vi "Sensor checking_try.vi"() -> ()   [LabVIEW 2016]
uses:
  <vilib>/rvi/Emulation/niFpgaGetClockAttributes.vi
  <vilib>/rvi/Emulation/niFpgaSctlEmulationGetInTimedLoop.vi
  <vilib>/rvi/Emulation/niFpgaEmulationReportErrorSimple.vi
  <vilib>/rvi/eio/common/nirviEmuTemplateMethod_errors.vi
  <vilib>/rvi/Emulation/niFpgaCriticalErrorInLSC.vi
  <vilib>/eio/EIONode/EIONode.xnode
panel:
  out "8 9":fxp<+/-,26,5> format="%#_6f"
  out "8 8":fxp<+/-,26,5> format="%#_6f"
  out "8 7":fxp<+/-,26,5> format="%#_6f"
  out "8 6":fxp<+/-,26,5> format="%#_6f"
  out "8 5":fxp<+/-,26,5> format="%#_6f"
  out "8 4":fxp<+/-,26,5> format="%#_6f"
  out "8 3":fxp<+/-,26,5> format="%#_6f"
  out "8 2":fxp<+/-,26,5> format="%#_6f"
  out "8 1":fxp<+/-,26,5> format="%#_6f"
  out "7 9":fxp<+/-,26,5> format="%#_6f"
  out "7 8":fxp<+/-,26,5> format="%#_6f"
  out "7 7":fxp<+/-,26,5> format="%#_6f"
  out "7 6":fxp<+/-,26,5> format="%#_6f"
  out "7 5":fxp<+/-,26,5> format="%#_6f"
  out "7 4":fxp<+/-,26,5> format="%#_6f"
  out "7 3":fxp<+/-,26,5> format="%#_6f"
  out "7 2":fxp<+/-,26,5> format="%#_6f"
  out "7 1":fxp<+/-,26,5> format="%#_6f"
  out "6 9":fxp<+/-,26,5> format="%#_6f"
  out "6 8":fxp<+/-,26,5> format="%#_6f"
  out "6 7":fxp<+/-,26,5> format="%#_6f"
  out "6 6":fxp<+/-,26,5> format="%#_6f"
  out "6 5":fxp<+/-,26,5> format="%#_6f"
  out "6 4":fxp<+/-,26,5> format="%#_6f"
  out "6 3":fxp<+/-,26,5> format="%#_6f"
  out "6 2":fxp<+/-,26,5> format="%#_6f"
  out "6 1":fxp<+/-,26,5> format="%#_6f"
  out "5 9":fxp<+/-,26,5> format="%#_6f"
  out "5 8":fxp<+/-,26,5> format="%#_6f"
  out "5 7":fxp<+/-,26,5> format="%#_6f"
  out "5 6":fxp<+/-,26,5> format="%#_6f"
  out "5 5":fxp<+/-,26,5> format="%#_6f"
  out "5 4":fxp<+/-,26,5> format="%#_6f"
  out "5 3":fxp<+/-,26,5> format="%#_6f"
  out "5 2":fxp<+/-,26,5> format="%#_6f"
  out "5 1":fxp<+/-,26,5> format="%#_6f"
  out "4 9":fxp<+/-,26,5> format="%#_6f"
  out "4 8":fxp<+/-,26,5> format="%#_6f"
  out "4 7":fxp<+/-,26,5> format="%#_6f"
  out "4 6":fxp<+/-,26,5> format="%#_6f"
  out "4 5":fxp<+/-,26,5> format="%#_6f"
  out "4 4":fxp<+/-,26,5> format="%#_6f"
  out "4 3":fxp<+/-,26,5> format="%#_6f"
  out "4 2":fxp<+/-,26,5> format="%#_6f"
  out "4 1":fxp<+/-,26,5> format="%#_6f"
  out "3 9":fxp<+/-,26,5> format="%#_6f"
  out "3 8":fxp<+/-,26,5> format="%#_6f"
  out "3 7":fxp<+/-,26,5> format="%#_6f"
  out "3 6":fxp<+/-,26,5> format="%#_6f"
  out "3 5":fxp<+/-,26,5> format="%#_6f"
  out "3 4":fxp<+/-,26,5> format="%#_6f"
  out "3 3":fxp<+/-,26,5> format="%#_6f"
  out "3 2":fxp<+/-,26,5> format="%#_6f"
  out "3 1":fxp<+/-,26,5> format="%#_6f"
  out "2 9":fxp<+/-,26,5> format="%#_6f"
  out "2 8":fxp<+/-,26,5> format="%#_6f"
  out "2 7":fxp<+/-,26,5> format="%#_6f"
  out "2 6":fxp<+/-,26,5> format="%#_6f"
  out "2 5":fxp<+/-,26,5> format="%#_6f"
  out "2 4":fxp<+/-,26,5> format="%#_6f"
  out "2 3":fxp<+/-,26,5> format="%#_6f"
  out "2 2":fxp<+/-,26,5> format="%#_6f"
  out "2 1":fxp<+/-,26,5> format="%#_6f"
  out "1 9":fxp<+/-,26,5>
  out "1 8":fxp<+/-,26,5>
  out "1 7":fxp<+/-,26,5>
  out "1 6":fxp<+/-,26,5>
  out "1 5":fxp<+/-,26,5>
  out "1 4":fxp<+/-,26,5>
  out "1 3":fxp<+/-,26,5>
  out "1 2":fxp<+/-,26,5> format="%#_6f"
  out "1 1":fxp<+/-,26,5> format="%#_6f"
  in  "8":bool
  in  "7":bool
  in  "6":bool
  in  "5":bool
  in  "4":bool
  in  "3":bool
  in  "2":bool
  in  "1":bool
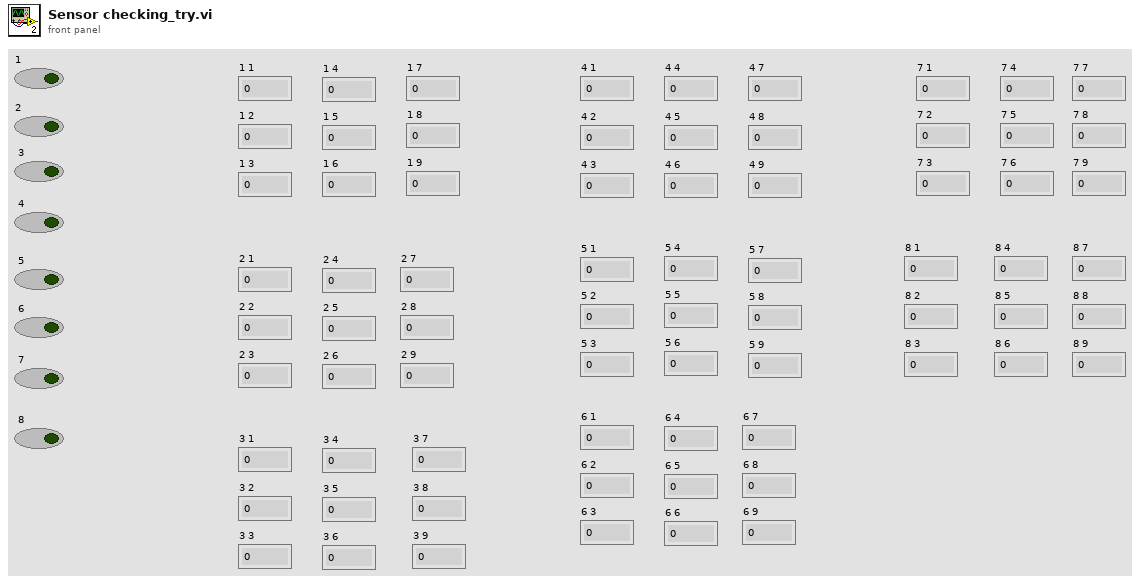
[diagram p1: front panel]
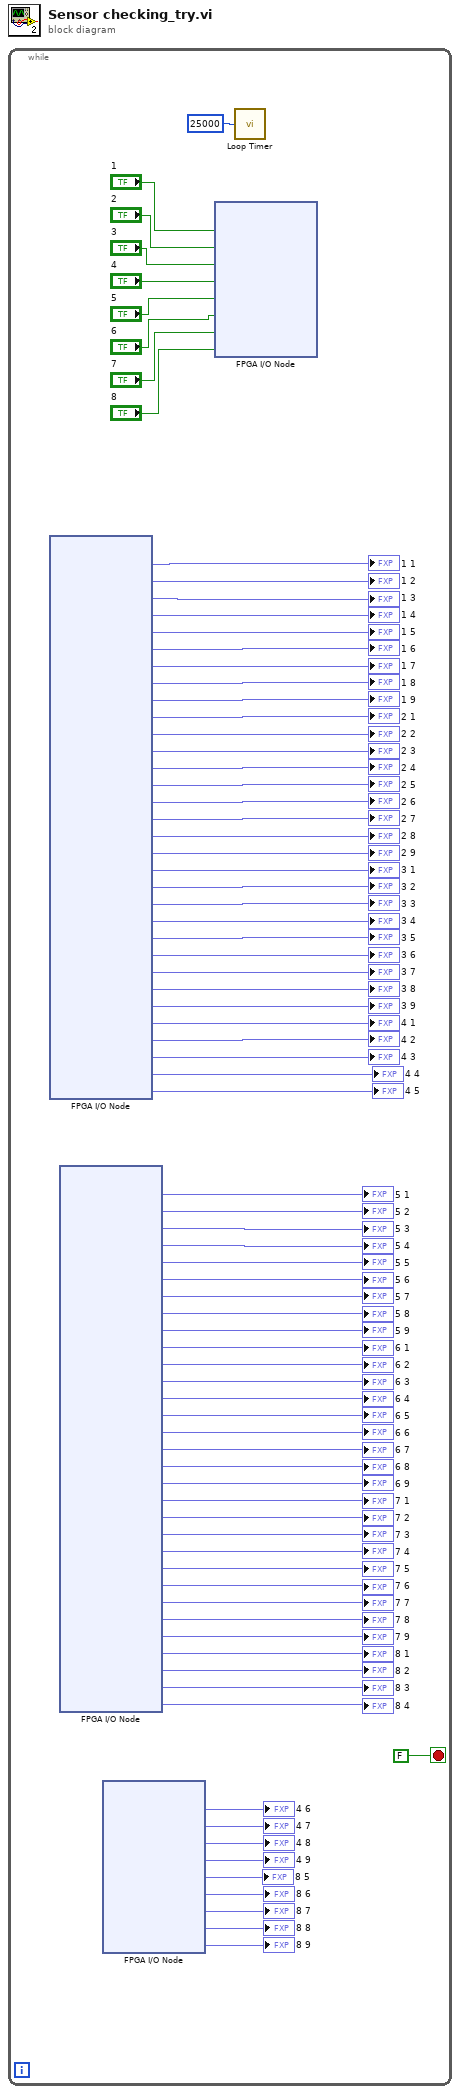
[diagram p0: block diagram]
diagram:
  n1 = while {
    stop <- FALSE stop-if-true
    n2 = xnode "FPGA I/O Node"() -> ("Mod1/AI0"=→"1 1":fxp<+/-,26,5>, "Mod1/AI1"=→"1 2":fxp<+/-,26,5>, "Mod1/AI2"=→"1 3":fxp<+/-,26,5>, "Mod1/AI3"=→"1 4":fxp<+/-,26,5>, "Mod1/AI4"=→"1 5":fxp<+/-,26,5>, "Mod1/AI5"=→"1 6":fxp<+/-,26,5>, "Mod1/AI6"=→"1 7":fxp<+/-,26,5>, "Mod1/AI7"=→"1 8":fxp<+/-,26,5>, "Mod1/AI8"=→"1 9":fxp<+/-,26,5>, "Mod1/AI9"=→"2 1":fxp<+/-,26,5>, "Mod1/AI10"=→"2 2":fxp<+/-,26,5>, "Mod1/AI11"=→"2 3":fxp<+/-,26,5>, "Mod1/AI12"=→"2 4":fxp<+/-,26,5>, "Mod1/AI13"=→"2 5":fxp<+/-,26,5>, "Mod1/AI14"=→"2 6":fxp<+/-,26,5>, "Mod1/AI15"=→"2 7":fxp<+/-,26,5>, "Mod1/AI16"=→"2 8":fxp<+/-,26,5>, "Mod1/AI17"=→"2 9":fxp<+/-,26,5>, "Mod1/AI18"=→"3 1":fxp<+/-,26,5>, "Mod1/AI19"=→"3 2":fxp<+/-,26,5>, "Mod1/AI20"=→"3 3":fxp<+/-,26,5>, "Mod1/AI21"=→"3 4":fxp<+/-,26,5>, "Mod1/AI22"=→"3 5":fxp<+/-,26,5>, "Mod1/AI23"=→"3 6":fxp<+/-,26,5>, "Mod1/AI24"=→"3 7":fxp<+/-,26,5>, "Mod1/AI25"=→"3 8":fxp<+/-,26,5>, "Mod1/AI26"=→"3 9":fxp<+/-,26,5>, "Mod1/AI27"=→"4 1":fxp<+/-,26,5>, "Mod1/AI28"=→"4 2":fxp<+/-,26,5>, "Mod1/AI29"=→"4 3":fxp<+/-,26,5>, "Mod1/AI30"=→"4 4":fxp<+/-,26,5>, "Mod1/AI31"=→"4 5":fxp<+/-,26,5>)  [unwired: 32 in, 32 out]
    n3 = xnode "FPGA I/O Node"() -> ("Mod8/AI0"=→"5 1":fxp<+/-,26,5>, "Mod8/AI1"=→"5 2":fxp<+/-,26,5>, "Mod8/AI2"=→"5 3":fxp<+/-,26,5>, "Mod8/AI3"=→"5 4":fxp<+/-,26,5>, "Mod8/AI4"=→"5 5":fxp<+/-,26,5>, "Mod8/AI5"=→"5 6":fxp<+/-,26,5>, "Mod8/AI6"=→"5 7":fxp<+/-,26,5>, "Mod8/AI7"=→"5 8":fxp<+/-,26,5>, "Mod8/AI8"=→"5 9":fxp<+/-,26,5>, "Mod8/AI9"=→"6 1":fxp<+/-,26,5>, "Mod8/AI10"=→"6 2":fxp<+/-,26,5>, "Mod8/AI11"=→"6 3":fxp<+/-,26,5>, "Mod8/AI12"=→"6 4":fxp<+/-,26,5>, "Mod8/AI13"=→"6 5":fxp<+/-,26,5>, "Mod8/AI14"=→"6 6":fxp<+/-,26,5>, "Mod8/AI15"=→"6 7":fxp<+/-,26,5>, "Mod8/AI16"=→"6 8":fxp<+/-,26,5>, "Mod8/AI17"=→"6 9":fxp<+/-,26,5>, "Mod8/AI18"=→"7 1":fxp<+/-,26,5>, "Mod8/AI19"=→"7 2":fxp<+/-,26,5>, "Mod8/AI20"=→"7 3":fxp<+/-,26,5>, "Mod8/AI21"=→"7 4":fxp<+/-,26,5>, "Mod8/AI22"=→"7 5":fxp<+/-,26,5>, "Mod8/AI23"=→"7 6":fxp<+/-,26,5>, "Mod8/AI24"=→"7 7":fxp<+/-,26,5>, "Mod8/AI25"=→"7 8":fxp<+/-,26,5>, "Mod8/AI26"=→"7 9":fxp<+/-,26,5>, "Mod8/AI27"=→"8 1":fxp<+/-,26,5>, "Mod8/AI28"=→"8 2":fxp<+/-,26,5>, "Mod8/AI29"=→"8 3":fxp<+/-,26,5>, "Mod8/AI30"=→"8 4":fxp<+/-,26,5>)  [unwired: 31 in, 31 out]
    n4 = xnode "FPGA I/O Node"() -> ("Mod5/AI0"=→"4 6":fxp<+/-,26,5>, "Mod5/AI1"=→"4 7":fxp<+/-,26,5>, "Mod5/AI2"=→"4 8":fxp<+/-,26,5>, "Mod5/AI3"=→"4 9":fxp<+/-,26,5>, "Mod5/AI30"=→"8 5":fxp<+/-,26,5>, "Mod1/AI20"=→"8 6":fxp<+/-,26,5>, "Mod1/AI21"=→"8 7":fxp<+/-,26,5>, "Mod1/AI22"=→"8 8":fxp<+/-,26,5>, "Mod1/AI23"=→"8 9":fxp<+/-,26,5>)  [unwired: 9 in, 9 out]
    n5 = xnode "FPGA I/O Node"("Mod6/DO0"="1", "Mod6/DO1"="2", "Mod6/DO2"="3", "Mod6/DO3"="4", "Mod6/DO4"="5", "Mod6/DO5"="6", "Mod6/DO6"="7", "Mod6/DO7"="8") -> ()  [unwired: 8 in, 8 out]
    n6 = call "Loop Timer"("Count(Ticks)"=u32 25000 ("Count(uSec)")) -> ()  [unwired: 1 out]
  }
